vi "Login Successful.vi"(0 "Login View in":refnum<class "Login View.lvclass">, 11 "error in (no error)":errorcluster) -> (4 "Login View out":refnum<class "Login View.lvclass">, 15 "error out":errorcluster)   [LabVIEW 2017, in "Login View.lvlib" / "Login View.lvclass"]
uses:
  Login View.lvclass
  User Manager Model/Type Definitions/Credentials.ctl
  Login View.lvclass/Login View.ctl
  User Manager Model/Type Definitions/User Manager Application Types.lvlib
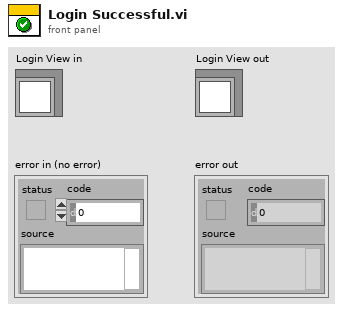
[diagram p1: front panel]
types:
  T1 = typedef "User Manager Application Types.lvlib/Credentials.ctl" = cluster{"Username":string, "Password":string}
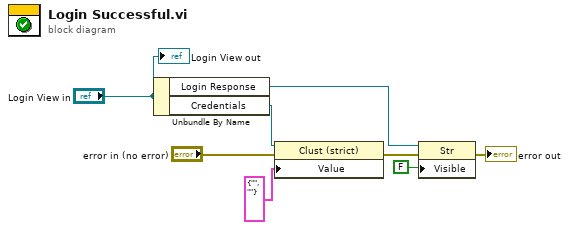
[diagram p0: block diagram]
diagram:
  n1 = Unbundle By Name("Login View in") -> ("Login Response"=w1:refnum<vi>, "Credentials"=w5:refnum<vi>)
  n2 = property on="Property Node" class="Clust (strict)"(reference=w5, error in="error in (no error)", "Value"=T1 {"Username"="", "Password"=""}) -> (error out=w2:errorcluster)  [unwired: 1 out]
  n3 = property on="Property Node" class="Str"(reference=w1, error in=w2, "Visible"=FALSE) -> (error out=→"error out":errorcluster)  [unwired: 1 out]
  "Login View out" <- "Login View in"
